vi "NaN_and_zeroFilter.vi"(3 "X":dbl, 4 "Y":dbl) -> (1 "NaNor0":bool)   [LabVIEW 2013]
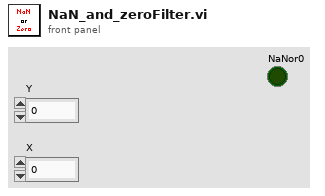
[diagram p1: front panel]
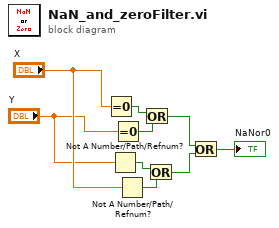
[diagram p0: block diagram]
diagram:
  n1 = Equal To 0?(x="X") -> (x = 0?=w5:bool)
  n2 = Not A Number/Path/Refnum?(number/path/refnum="Y") -> (NaN/Path/Refnum?=w2:bool)
  n3 = Equal To 0?(x="Y") -> (x = 0?=w4:bool)
  n4 = Not A Number/Path/Refnum?(number/path/refnum="X") -> (NaN/Path/Refnum?=w3:bool)
  n5 = Or(x=w5, y=w4) -> (x .or. y?=w7:bool)
  n6 = Or(x=w2, y=w3) -> (x .or. y?=w6:bool)
  n7 = Or(x=w7, y=w6) -> (x .or. y?=→"NaNor0":bool)
